vi "DI B Config.vi"(8 "Device Inputs":dbl[](array[numeric]), 10 "B Config FIFO Indexes":T5, 11 "B Configuration in":T1 {"Pump Zener Voltage [V]" min=0 max=240 format="%#_13g"; "DI Zener Voltage [V]" min=0 max=100 format="%#_13g"; "Boost Clamp [V]" min=0 max=220 format="%#_13g"; "Boost Voltage [V]" min=0 max=220 format="%#_13g"}) -> (3 "B Configuration":T3 {"Pump Zener Voltage [V]" min=0 max=240 format="%#_13g"; "DI Zener Voltage [V]" min=0 max=100 format="%#_13g"; "Boost Clamp [V]" min=0 max=220 format="%#_13g"; "Boost Voltage [V]" min=0 max=220 format="%#_13g"})   [LabVIEW 2016, in "DCM Engine.lvlib"]
uses:
  DCM Engine.lvlib
  Built/DCM Classes Packed/Pharlap/C/DCM-Classes.lvlibp/DCM/Rev0/RT/Configuration.ctl
  Built/DCM Classes Packed/Pharlap/C/DCM-Classes.lvlibp/1abvi3w/vi.lib/Powertrain Controls/Device Drivers/DCM/Rev0/FPGA/DI - Bank Configuration.ctl
  <vilib>/Powertrain Controls/Device Drivers/DCM/Rev0/RT/Configuration.ctl
  <vilib>/Powertrain Controls/Device Drivers/DCM/Rev0/FPGA/DI - Bank Configuration.ctl
  Built/DCM Classes Packed/Pharlap/C/DCM-Classes.lvlibp/1abvi3w/vi.lib/Powertrain Controls/Device Drivers/DCM/Rev0/FPGA/DCM - FPGA.lvlib
  Built/DCM Classes Packed/Pharlap/C/DCM-Classes.lvlibp/DCM/Rev0/RT/DCM - RT.lvclass
  <vilib>/Powertrain Controls/Device Drivers/DCM/Rev0/FPGA/DCM - FPGA.lvlib
  <vilib>/Powertrain Controls/Device Drivers/DCM/Rev0/RT/DCM - RT.lvclass
panel:
  # "Voltage [DV]"
  # "Voltage [V]"
  # "Voltage [DV]"
  # "Voltage [V]"
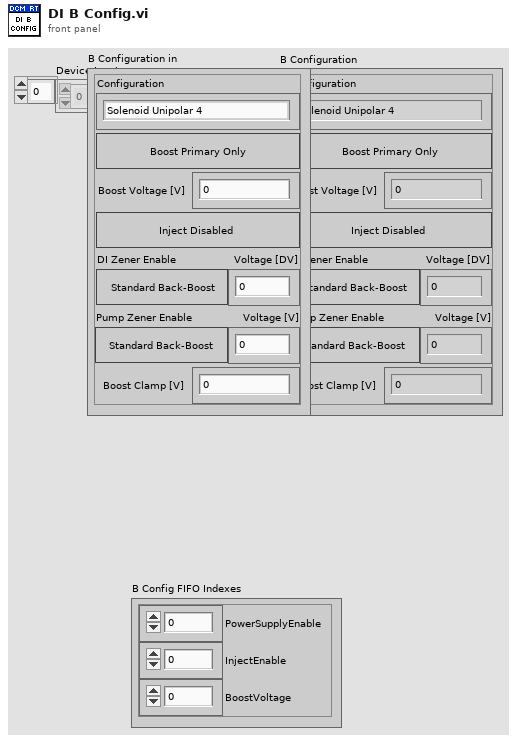
[diagram p1: front panel]
types:
  T1 = typedef "DCM - RT.lvclass/Configuration.ctl" = cluster{"Configuration":T2, "Power Supply Enable":bool, "Boost Voltage [V]":sgl, "Inject Enable":bool, "DI Zener Enable":bool, "DI Zener Voltage [V]":sgl, "Pump Zener Enable":bool, "Pump Zener Voltage [V]":sgl, "Boost Clamp [V]":sgl}
  T2 = typedef "DCM - FPGA.lvlib/DI - Bank Configuration.ctl" = enum8{"Solenoid Unipolar 4", "Solenoid Unipolar 7 (Muxed)", "Solenoid Unipolar 8 (Muxed)", "Solenoid Bipolar 2", "Solenoid Bipolar 3 (Muxed)", "Piezo Unipolar 2", "Piezo Unipolar 3 (Muxed)", "Piezo Unipolar 4 (Muxed)", "Piezo Bipolar 2", "Piezo Bipolar 3 (Muxed)"}
  T3 = typedef "DCM-Classes.lvlibp/DCM - RT.lvclass/Configuration.ctl" = cluster{"Configuration":T4, "Power Supply Enable":bool, "Boost Voltage [V]":sgl, "Inject Enable":bool, "DI Zener Enable":bool, "DI Zener Voltage [V]":sgl, "Pump Zener Enable":bool, "Pump Zener Voltage [V]":sgl, "Boost Clamp [V]":sgl}
  T4 = typedef "DCM-Classes.lvlibp/DCM - FPGA.lvlib/DI - Bank Configuration.ctl" = enum8{"Solenoid Unipolar 4", "Solenoid Unipolar 7 (Muxed)", "Solenoid Unipolar 8 (Muxed)", "Solenoid Bipolar 2", "Solenoid Bipolar 3 (Muxed)", "Piezo Unipolar 2", "Piezo Unipolar 3 (Muxed)", "Piezo Unipolar 4 (Muxed)", "Piezo Bipolar 2", "Piezo Bipolar 3 (Muxed)"}
  T5 = cluster{"PowerSupplyEnable":i32, "InjectEnable":i32, "BoostVoltage":i32}
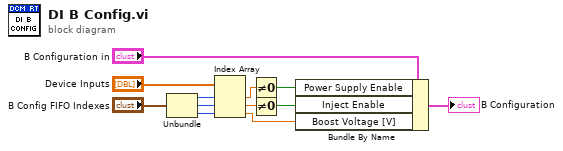
[diagram p0: block diagram]
diagram:
  n1 = Unbundle("B Config FIFO Indexes") -> ("PowerSupplyEnable"=w7:i32, "InjectEnable"=w6:i32, "BoostVoltage"=w5:i32)
  n2 = Index Array(array="Device Inputs", index #1=w7, index #2=w6, index #3=w5) -> (element #1=w10:dbl, element #2=w4:dbl, element #3=w3:dbl)
  n3 = Not Equal To 0?(x=w10) -> (x != 0?=w11:bool)
  n4 = Not Equal To 0?(x=w4) -> (x != 0?=w2:bool)
  n5 = Bundle By Name(cluster="B Configuration in", "Power Supply Enable"=w11, "Inject Enable"=w2, "Boost Voltage [V]"=w3) -> (→"B Configuration":T1)
